vi "server.vi"(8 "error in (no error)":errorcluster, 11 "Port (5555)":i32=5555) -> (0 "error out":errorcluster)   [LabVIEW 2020, in "splash_screen.lvclass"]
uses:
  splash_screen.lvclass
  <vilib>/addons/zeromq/socket_type.ctl
  <vilib>/addons/zeromq/zmq_context.lvclass
  <vilib>/addons/zeromq/zeromq.lvlib
  <vilib>/addons/zeromq/zmq_socket.lvclass
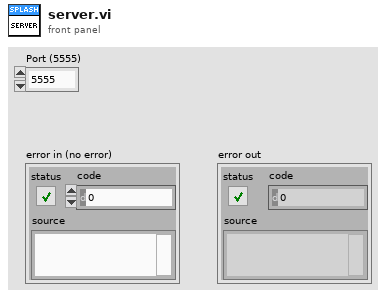
[diagram p1: front panel]
types:
  T1 = typedef "zeromq.lvlib/socket_type.ctl" = enum8{"ZMQ_PAIR", "ZMQ_PUB", "ZMQ_SUB", "ZMQ_REQ", "ZMQ_REP", "ZMQ_DEALER", "ZMQ_ROUTER", "ZMQ_PULL", "ZMQ_PUSH", "ZMQ_XPUB", "ZMQ_XSUB", "ZMQ_STREAM", "ZMQ_SERVER", "ZMQ_CLIENT", "ZMQ_RADIO", "ZMQ_DISH", "ZMQ_GATHER", "ZMQ_SCATTER", "ZMQ_DGRAM"}
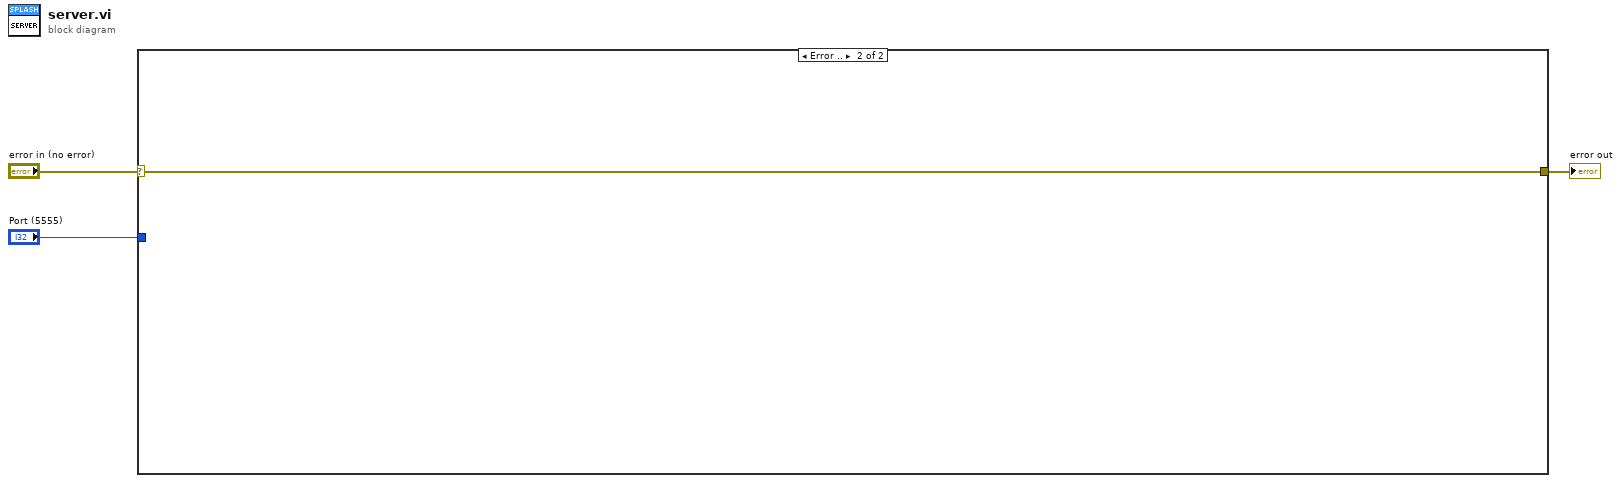
[diagram p0: block diagram]
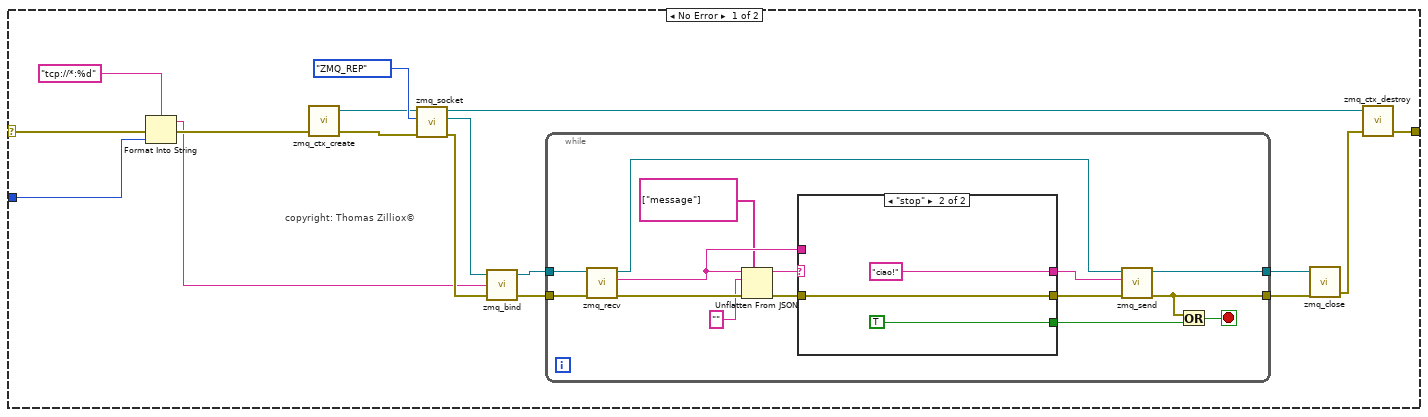
[diagram p2: hidden frame]
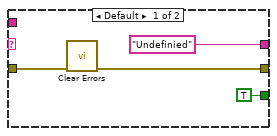
[diagram p3: hidden frame]
diagram:
  n1 = case shown="Error .." "error in (no error)" {
    selector: "error in (no error)" -> [w4 w43]
    tunnel: [w20 w43] -> w3
    tunnel: "Port (5555)" -> [w7 _]
    frame No Error {
      # "copyright: Thomas Zilliox©"
      n2 = Format Into String(format string="tcp://*:%d" ("endpoint"), error in=w4, w7) -> (resulting string=w5:string, error out=w8:errorcluster)  [unwired: 1 in]
      n3 = call <vilib>:"zmq_ctx_create.vi"("error in"=w8) -> ("error out"=w10:errorcluster, "context out"=w9:refnum<class "zmq_context.lvclass">)  [unwired: 3 in]
      n4 = call <vilib>:"zmq_socket.vi"("error in"=w10, "socket type"=socket_type."ZMQ_REP", "context in"=w9) -> ("error out"=w14:errorcluster, "socket out"=w13:refnum<class "zmq_socket.lvclass">, "context out"=w12:refnum<class "zmq_context.lvclass">)  [unwired: 2 in]
      n5 = call <vilib>:"zmq_bind.vi"("error in"=w14, "endpoint"=w5, "socket in"=w13) -> ("error out"=w16:errorcluster, "socket out"=w15:refnum<class "zmq_socket.lvclass">)  [unwired: 1 in]
      n6 = while {
        tunnel: w15 -> [w35]
        tunnel: w16 -> [w34]
        tunnel: [w32] -> w17
        tunnel: [w31] -> w18
        stop <- w30 stop-if-true
        n7 = call <vilib>:"zmq_recv.vi"("error in"=w34, "socket in"=w35) -> ("error out"=w27:errorcluster, "data"=w23:string, "socket out"=w33:refnum<class "zmq_socket.lvclass">)  [unwired: 3 in, 2 out]
        n8 = Unflatten From JSON(path=string[] ["message"], JSON string=w23, type and defaults="", error in (no error)=w27) -> (value=w25:string, error out=w26:errorcluster)  [unwired: 3 in]
        n9 = case shown="\"stop\"" w25 {
          tunnel: [w36 w42] -> w29
          tunnel: w26 -> [w39 w42]
          tunnel: [TRUE TRUE] -> w28
          tunnel: ["Undefinied" ("data") "ciao!" ("data")] -> w22
          tunnel: w23 -> [_ _]
          frame Default {
            n10 = call <vilib>:"Clear Errors.vi"("error in (no error)"=w39) -> ("error out"=w36:errorcluster)  [unwired: 5 in, 1 out]
          }
          frame "stop" {
          }
        }
        n11 = call <vilib>:"zmq_send.vi"("error in"=w29, "data"=w22, "socket in"=w33) -> ("error out"=w31:errorcluster, "socket out"=w32:refnum<class "zmq_socket.lvclass">)  [unwired: 4 in]
        n12 = Or(x=w31, y=w28) -> (x .or. y?=w30:bool)
      }
      n13 = call <vilib>:"zmq_close.vi"("error in"=w18, "socket"=w17) -> ("error out"=w19:errorcluster)  [unwired: 3 in]
      n14 = call <vilib>:"zmq_ctx_destroy.vi"("error in"=w19, "context in"=w12) -> ("error out"=w20:errorcluster)  [unwired: 3 in]
    }
    frame Error {
    }
  }
  "error out" <- w3
